vi "getTimeStamp.vi"() -> (2 "nsecs":i32, 3 "secs":i32, 4 "ROS Time":cluster{"secs":i32, "nsecs":i32})   [LabVIEW 2015]
doc: "Returns the current time stamp in ROS time"
uses:
  vi.lib/Utility/miscctls.llb/LVDateTimeRec.ctl
panel:
  out "days since epoch":i32
  out "date time rec":T1
  out "current time":timestamp
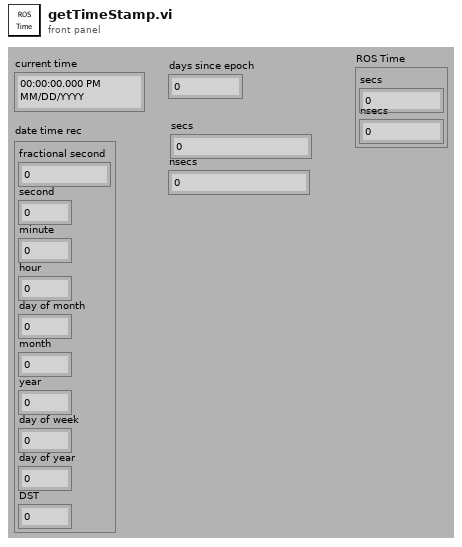
[diagram p1: front panel]
types:
  T1 = typedef "LVDateTimeRec.ctl" = cluster{"fractional second":dbl, "second":i32, "minute":i32, "hour":i32, "day of month":i32, "month":i32, "year":i32, "day of week":i32, "day of year":i32, "DST":i32}
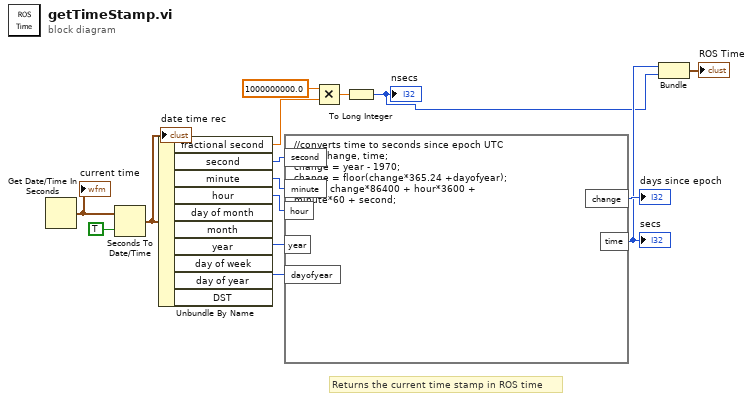
[diagram p0: block diagram]
diagram:
  # "Returns the current time stamp in ROS time"
  n1 = Get Date/Time In Seconds() -> (seconds since 1Jan1904=w6:timestamp)
  "current time" <- w6
  n2 = Seconds To Date/Time(time stamp (now)=w6, to UTC (F)=TRUE) -> (date time rec=w13:T1)
  "date time rec" <- w13
  n3 = Unbundle By Name(w13) -> ("fractional second"=w5:dbl, "second"=w11:i32, "minute"=w10:i32, "hour"=w9:i32, "year"=w7:i32, "day of year"=w8:i32)  [unwired: 4 out]
  n4 = formula code="//converts time to seconds since epoch UTC\nint32 change, time;\nchange = year - 1970;\nchange = floor(change*365.24 +dayofyear);\ntime = change*86400 + hour*3600 +\nminute*60 + second;"("year"=w7, "dayofyear"=w8, "hour"=w9, "minute"=w10, "second"=w11) -> ("change"=→"days since epoch":i32, "time"=w3:i32)
  "secs" <- w3
  n5 = Multiply(x=1000000000.0 ("y"), y=w5) -> (x*y=w15:dbl)
  n6 = To Long Integer(number=w15) -> (32bit integer=w2:i32)
  "nsecs" <- w2
  n7 = Bundle(w3, w2) -> (→"ROS Time":cluster{i32, i32})  [unwired: 1 in]
